vi "make_path_absolute.vi"(8 "error in (no error)":errorcluster, 11 "relative path":string) -> (0 "error out":errorcluster, 3 "absolute path":path)   [LabVIEW 2010]
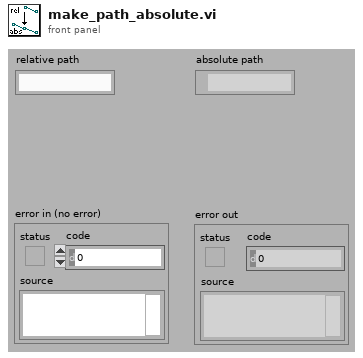
[diagram p1: front panel]
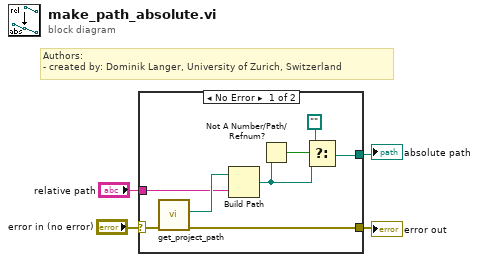
[diagram p0: block diagram]
diagram:
  # "Authors: \n- created by: Dominik Langer, University of Zurich, Switzerland"
  n1 = case shown="No Error" "error in (no error)" {
    selector: "error in (no error)" -> [w12 w13]
    tunnel: [w9 w13] -> w3
    tunnel: "relative path" -> [w10 _]
    tunnel: [w5 _] -> w1
    frame No Error {
      n2 = call "get_project_path.vi"("error in (no error)"=w12) -> ("error out"=w9:errorcluster, "helioscan path"=w11:path)  [unwired: 9 in]
      n3 = Build Path(base path=w11, name or relative path=w10) -> (appended path=w6:path)
      n4 = Not A Number/Path/Refnum?(number/path/refnum=w6) -> (NaN/Path/Refnum?=w8:bool)
      n5 = Select(t=path "", s=w8, f=w6) -> (s? t:f=w5:path)
    }
    frame Error {
    }
  }
  "absolute path" <- w1
  "error out" <- w3
